vi "unmixing 2color images.vi"(4 "parameters":T1, 5 "ch2":dbl[][](array[numeric]), 8 "ch1":dbl[][](array[numeric])) -> (0 "unmixed ch2":dbl[][](array[numeric]), 3 "unmixed ch1":dbl[][](array[numeric]))   [LabVIEW 2018]
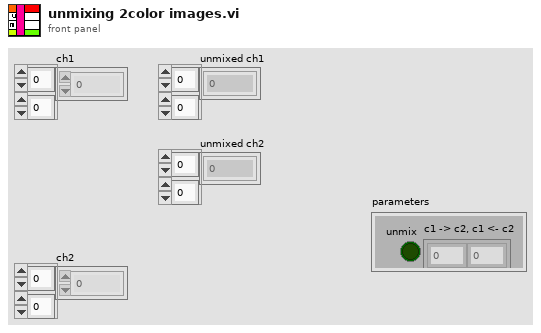
[diagram p1: front panel]
types:
  T1 = cluster{"c1 -> c2, c1 <- c2":dbl[], "unmix":bool}
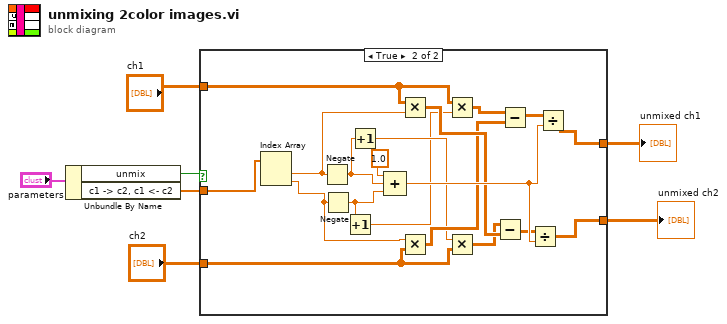
[diagram p0: block diagram]
diagram:
  n1 = Unbundle By Name("parameters") -> ("unmix"=w2:bool, "c1 -> c2, c1 <- c2"=w1:dbl[])
  n2 = case shown="True" w2 {
    tunnel: [w8 w28] -> w7
    tunnel: [w9 w27] -> w6
    tunnel: "ch1" -> [w9 w26]
    tunnel: "ch2" -> [w8 w22]
    tunnel: w1 -> [_ w10]
    frame False {
    }
    frame True {
      n3 = Index Array(array=w10) -> (element #1=w12:dbl, element #2=w11:dbl)  [unwired: 2 in]
      n4 = Negate(x=w12) -> (-x=w15:dbl)
      n5 = Negate(x=w11) -> (-x=w14:dbl)
      n6 = Increment(x=w14) -> (x+1=w16:dbl)
      n7 = Increment(x=w15) -> (x+1=w17:dbl)
      n8 = Compound Arithmetic op=ADD(1.0 ("value"), w15, w14) -> (w25:dbl)
      n9 = Multiply(x=w26, y=w12) -> (x*y=w21:dbl[][])
      n10 = Multiply(x=w11, y=w22) -> (x*y=w19:dbl[][])
      n11 = Multiply(x=w26, y=w16) -> (x*y=w18:dbl[][])
      n12 = Multiply(x=w17, y=w22) -> (x*y=w20:dbl[][])
      n13 = Subtract(x=w20, y=w21) -> (x-y=w24:dbl[][])
      n14 = Subtract(x=w18, y=w19) -> (x-y=w23:dbl[][])
      n15 = Divide(x=w24, y=w25) -> (x/y=w28:dbl[][])
      n16 = Divide(x=w23, y=w25) -> (x/y=w27:dbl[][])
    }
  }
  "unmixed ch2" <- w7
  "unmixed ch1" <- w6
